vi "GetNI_PassData.vi"(0 "Digitizer Settings":T1={"Digitizer delay (us) "=0.0, "rf points per line"=2048, "lines per plane"=128, "Samp Rate (Hz)"=100000000.0, "Additional dig delay (us)"=0.0, "Voltage Scale"=0.4, "Pre-Looks"=0, "Offset delay (us)"=0.0, "bits A/D"=8, "Avg Num"=1, "DigTimeOut"=5.0, "Rel Dig Delay"=0.0, "Dig Ch"=0, "LeCroyCluster"={"LeCroy Channels"=[TRUE, FALSE, FALSE, FALSE], "LC read pt offset"=0.0, "Sweep Avg"=FALSE}, "Main Digitizer"=enum."NI Digitizer", "Dig Config"=enum."Single channel", "Digitizer ID Cluster"={"Acqiris/Alazar/SP ID"=[], "NI Instr Handles"=[], "LeCroy VISA"="", "GaGe Handle"={"Handle"=0, "Sample size"=0, "Resolution"=0, "Offset"=0, "Channels"=0, "Boards"=0}, "ATS Ref"="ATS9350", "Acqiris Address"=["PCI::INSTR0"], "ADQRef"=refnum, "adq_cu_ptr"=refnum}, "Trigger Settings"={"Trig Source"=1, "Trig Coupling"=0, "Trig Slope"=0, "Level (mV)"=1500.0}, "Bulk Acq"=FALSE, "Bulk Start Indexes"=[], "Data Ref RF"=refnum, "NI ID/Channel"=[], "Total Dig CH"=1, "Xtra Ann Trig delay (us)"=10.0, "Fix Z Delay?"=FALSE, "One Way Transmission?"=FALSE, "Data Ref Log"=refnum} {"Trigger Settings"."Trig Slope" items=["Positive", "Negative"]; "Trigger Settings"."Level (mV)" format="%.2f"; "Trigger Settings"."Trig Coupling" items=["DC 1 MOhm", "AC 1 MOhm", "DC 50 Ohm", "AC 50 Ohm"]; "Trigger Settings"."Trig Source" items=["Chan 1", "External"]; "Rel Dig Delay" format="%.2f"; "DigTimeOut" format="%.2f"; "Avg Num" min=1; "Offset delay (us)" format="%.2f"; "Additional dig delay (us)" format="%.2f"; "Digitizer delay (us)" format="%.2f"}, 3 "NI Card":refnum<k15>, 7 "errorin":errorcluster, 8 "File Array":string[](array[string]), 15 "Reverse?":bool) -> (17 "Raw VGain (scale)":dbl, 18 "Gain Array":T5(array[cluster]), 20 "Array":i16[][][](array[numeric]), 21 "VGain (dB)":dbl, 27 "error out":errorcluster)   [LabVIEW 2022 SP3]
uses:
  -DigitizerRoutines/DigitizerSettings.ctl
  -DigitizerRoutines/Digitizer.ctl
  -DigitizerRoutines/DigConfig.ctl
  -DigitizerRoutines/DigitizerID.ctl
  C:/Windows/System32/ADQAPI_dotNet_helper.dll
  <instrlib>/niScope/Acquire/Fetch/niScope Multi Fetch Binary 8.vi
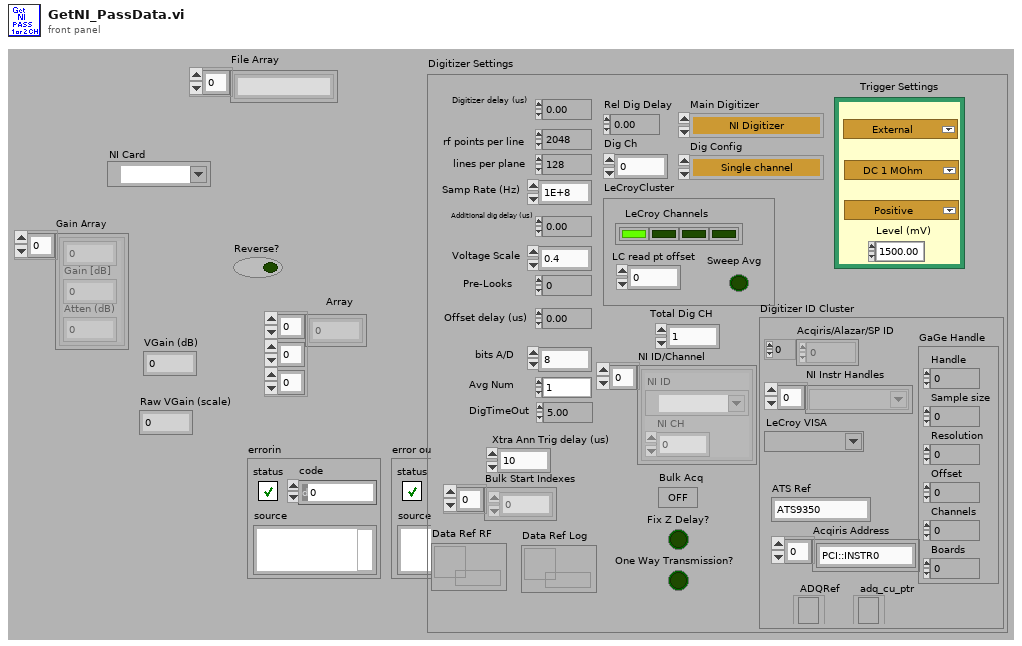
[diagram p1: front panel]
types:
  T1 = typedef "DigitizerSettings.ctl" = cluster{"Digitizer delay (us) ":dbl, "rf points per line":i32, "lines per plane":i32, "Samp Rate (Hz)":dbl, "Additional dig delay (us)":dbl, "Voltage Scale":dbl, "Pre-Looks":i32, "Offset delay (us)":dbl, "bits A/D":i8, "Avg Num":i32, "DigTimeOut":sgl, "Rel Dig Delay":sgl, "Dig Ch":i32, "LeCroyCluster":cluster{"LeCroy Channels":bool[], "LC read pt offset":dbl, "Sweep Avg":bool}, "Main Digitizer":T2, "Dig Config":T3, "Digitizer ID Cluster":T4, "Trigger Settings":cluster{"Trig Source":u16, "Trig Coupling":u16, "Trig Slope":u16, "Level (mV)":dbl}, "Bulk Acq":bool, "Bulk Start Indexes":i32[], "Data Ref RF":refnum<data-value>, "NI ID/Channel":cluster{"NI ID":refnum<k15>, "NI CH":i32}[], "Total Dig CH":i32, "Xtra Ann Trig delay (us)":dbl, "Fix Z Delay?":bool, "One Way Transmission?":bool, "Data Ref Log":refnum<data-value>}
  T2 = typedef "Digitizer.ctl" = enum16{"Acqiris Digitizer", "NI Digitizer", "LeCroy", "GaGe", "AlazarTech", "No Digitizer", "Teledyne"}
  T3 = typedef "DigConfig.ctl" = enum16{"Single channel", "2 Chans w/ 2 Acqiris", "2 Chans w/ 1 Acqiris", "5-CH Pulser New", "5-CH pulser w/ ann array", "5-pass style ann array", "Empty"}
  T4 = typedef "DigitizerID.ctl" = cluster{"Acqiris/Alazar/SP ID":u32[], "NI Instr Handles":refnum<k15>[], "LeCroy VISA":refnum<visa-resource-name>, "GaGe Handle":cluster{"Handle":u32, "Sample size":u32, "Resolution":i32, "Offset":i32, "Channels":u32, "Boards":u32}, "ATS Ref":string, "Acqiris Address":string[], "ADQRef":refnum<k24>, "adq_cu_ptr":refnum<k24>}
  T5 = cluster{sgl, "Gain [dB]  ":sgl, "Atten (dB)":sgl}[]
  T6 = cluster{"actualSamples":i32, "absoluteInitialX":dbl, "relativeInitialX":dbl, "xIncrement":dbl, "offset":dbl, "gain":dbl, "reserved1":dbl, "reserved2":dbl}[]
  T7 = cluster{"actualSamples":i32, "absoluteInitialX":dbl, "relativeInitialX":dbl, "xIncrement":dbl, "offset":dbl, "gain":dbl, "reserved1":dbl, "reserved2":dbl}
  T8 = cluster{sgl, "Gain [dB]  ":sgl, "Atten (dB)":sgl}
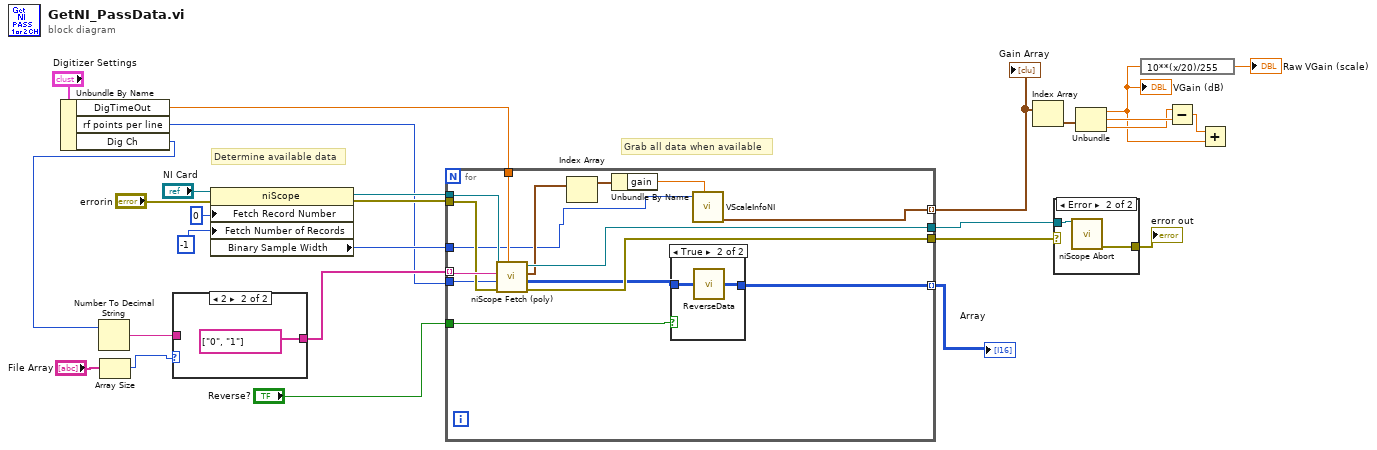
[diagram p0: block diagram]
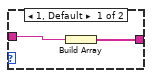
[diagram p3: hidden frame]
diagram:
  # "Grab all data when available"
  # "Determine available data"
  n1 = Unbundle By Name("Digitizer Settings") -> ("DigTimeOut"=w3:sgl, "rf points per line"=w4:i32, "Dig Ch"=w1:i32)
  n2 = Number To Decimal String(number=w1) -> (decimal integer string=w14:string)  [unwired: 1 out]
  n3 = Array Size(array="File Array") -> (size(s)=w13:i32)
  n4 = case shown="2" w13 {
    tunnel: [w29 string[] ["0", "1"] ("File Array")] -> w15
    tunnel: w14 -> [w28 _]
    frame 1, Default {
      n5 = Build Array(w28) -> (w29:string[])
    }
    frame 2 {
    }
  }
  n6 = property class="niScope"(reference="NI Card", error in="errorin", "Fetch Record Number"=0 ("Fetch:Fetch Record Number"), "Fetch Number of Records"=-1 ("Fetch:Fetch Number of Records")) -> (reference out=w19:refnum<k15>, error out=w18:errorcluster, "Binary Sample Width"=w6:i32)
  n7 = for {
    tunnel: [w40] -> w8
    tunnel: w15 -> [w45] mode=indexing
    tunnel: w3 -> [w39]
    tunnel: w19 -> [w44]
    tunnel: w18 -> [w43]
    tunnel: w4 -> [w42]
    tunnel: [w41] -> w9
    tunnel: [w33] -> w10 mode=indexing
    tunnel: "Reverse?" -> [w34]
    tunnel: w6 -> [w32]
    tunnel: [w31] -> w5 mode=indexing
    n8 = call-poly <instrlib>:"niScope Fetch (poly).vi"("timeout"=w39, "error in"=w43, "numSamples"=w42, "channels"=w45, "instrument handle"=w44) -> ("error out"=w41:errorcluster, "wfm"=w35:i8[][], "wfm info"=w38:T6, "instrument handle out"=w40:refnum<k15>)  [unwired: 3 out]
    n9 = Index Array(array=w38) -> (element=w37:T7)  [unwired: 1 in]
    n10 = Unbundle By Name(w37) -> ("gain"=w36:dbl)
    n11 = case shown="True" w34 {
      tunnel: w35 -> [w46 w48]
      tunnel: [w46 w47] -> w31
      frame False {
      }
      frame True {
        n12 = call "ReverseData.vi"("Array in"=w48) -> ("Array out"=w47:i16[][])
      }
    }
    n13 = call "VScaleInfoNI.vi"("A/D bits"=w32, "gain"=w36) -> ("Voltage Scale"=w33:T8)  [unwired: 5 in, 3 out]
  }
  "Gain Array" <- w10
  "Array" <- w5
  n14 = Index Array(array=w10) -> (element=w22:T8)  [unwired: 1 in]
  n15 = case shown="Error" w9 {
    selector: w9 -> [w49 _]
    tunnel: [w49 w51] -> w21
    tunnel: w8 -> [_ w50]
    frame No Error {
    }
    frame Error {
      n16 = call <instrlib>:"niScope Abort.vi"("instrument handle"=w50) -> ("error out"=w51:errorcluster)  [unwired: 1 in, 13 out]
    }
  }
  "error out" <- w21
  n17 = Unbundle(w22) -> (w23:sgl, "Gain [dB]"=w25:sgl, "Atten (dB)"=w24:sgl)
  "VGain (dB)" <- w23
  n18 = expression code="10**(x/20)/255"(w23) -> (→"Raw VGain (scale)":sgl)
  n19 = Subtract(x=w24, y=w25) -> (x-y=w26:sgl)
  n20 = Add(x=w26, y=w23) -> ()  [unwired: 1 out]
